vi "SR830Monitor.vi"(0 "Lock-in Reference":u16(ring) items=["Lock-in 1", "Lock-in 2", "Lock-in 3"]) -> ()   [LabVIEW 2019]
doc: "This VI is an example of storing and recovering data from the SR830 data buffers .\nDATA STORAGE RATE specifes the rate at which data is added to the data buffers .\nSCAN LENGTH specifies the approximate length of the data acquisition scan is seconds .\nPLOT GRAPH, PLOT CH 1 DATA and PLOT CH 2 DATA specify if the respective graphs will be displayed .\nAfter data storage is completed , the channel 1 and channel 2 points are downloaded from the instrument to the CH 1 POINTS and CH 2 POINTS arrays respectively . \nSince data recovered (using the SR830 receive message.vi) is in the string format , this VI requires a considerable amount of time to format the data into an array of floating point numbers . A quicker way would be to store the string in a file and use a CIN to speed up the process ."
uses:
  Utility/Monitor Communication/SR830/SR830-Cluster.ctl
  Utility/Monitor Communication/SR830/SR830-Settings-Cluster.ctl
  Global/Global Variables/Data_Display_global.vi
  Instrument_Setup.vi
  Utility/Monitor Communication/sub-vis/SR830_Open_Queue.vi
  Utility/Monitor Communication/sub-vis/SR830-2_Open_Queue.vi
  Utility/Monitor Communication/sub-vis/SR830-3_Open_Queue.vi
  Utility/Monitor Communication/sub-vis/SR830_Check_Queue.vi
panel:
  out "Sensitivity 2":i16(ring)=15 items=["2 nV", "5 nV", "10 nV", "20 nV", "50 nV", "100 nV", "200 nV", "500 nV", "1 µV", "2 µV", "5 µV", "10 µV", "20 µV", "50 µV", "100 µV", "200 µV", "500 µV", "1 mV", "2 mV", "5 mV", "10 mV", "20 mV", "50 mV", "100 mV", "200 mV", "500 mV", "1 V", ""]
  out "SR830-3 Settings":T1={"VISA"="GPIB0::17::INSTR", "Display Channel 2"={" display"=0, " ratio"=0, "output"=1}, "Display Channel 1"={" display"=0, " ratio"=0, "output"=1}, "Time constant"={"time constant\n(10 µs : 0) "=12, "slope (6 dB/oct)"=3}, "Sensitivity"={"sensitivity\n2nV/fA"=0, "dyn reserve\n(low noise:2)"=2, "ref. phase"=0.0, "automeasure"=FALSE}, "Offset - Expand."={"Expand (0: x1)"=0, "Offset/Expand Parameter (1: X)"=1, "Manual Offset (0)"=0.0}, "Reference"={"ref. source"=TRUE, "osc.harm# "=1, "osc. freq"=22.08, "osc. ampl."=5.0, "ref. trigger"=0}, "Lock In 1 sync"={"sync filter"=FALSE, "line filter\n(off:0)"=0}, "Lock In 1 input"={"input"=1, "ground"=FALSE, "couple"=TRUE}} {"Lock In 1 input"."input" items=["A", "A-B", "I (1 M gain)", "I (100 M gain)"]; "Lock In 1 sync"."line filter\n(off:0)" items=["OFF", "line", "2 x line", "both"]; "Reference"."ref. trigger" items=["sine", "pos edge", "neg edge"]; "Reference"."osc.harm#" min=1 max=19999; "Reference"."osc. ampl." format="%.3f"; "Reference"."osc. freq" format="%.3f"; "Offset - Expand."."Offset/Expand Parameter (1: X)" items=["X"=1, "Y"=2, "R"=3]; "Offset - Expand."."Expand (0: x1)" items=["x1", "x10", "x100"]; "Sensitivity"."sensitivity\n2nV/fA" items=["2 nV/fA", "5 nV/fA", "10 nV/fA", "20 nV/fA", "50 nV/fA", "100 nV/fA", "200 nV/fA", "500 nV/fA", "1 µV /pA", "2 µV/pA", "5 µV/pA", "10 µV/pA", "20 µV/pA", "50 µV/pA", "100 µV/pA", "200 µV/pA", "500 µV/pA", "1 mV/nA", "2 mV/nA", "5 mV/nA", "10 mV/nA", "20 mV/nA", "50 mV/nA", "100 mV/nA", "200 mV/nA", "500 mV/nA", "1 V/µA"]; "Sensitivity"."dyn reserve\n(low noise:2)" scale=0.0..2.0 scale format="%.2f"; "Sensitivity"."ref. phase" format="%.2f"; "Time constant"."slope (6 dB/oct)" items=["6 dB/oct", "12 dB/oct", "18 dB/oct", "24 dB/oct"]; "Time constant"."time constant\n(10 µs : 0)" items=["10 µs", "30 µs", "100 µs", "300 µs", "1 ms", "3 ms", "10 ms", "30 ms", "100 ms", "300 ms", "1 s", "3 s", "10 s", "30 s", "100 s", "300 s", "1 ks", "3 ks", "10 ks", "30 ks"]; "Display Channel 1"."output" items=["display", "X"]; "Display Channel 1"."ratio" items=["none", "aux in 1", "aux in 2"]; "Display Channel 1"."display" items=["X", "R", "X Noise", "Aux In 1", "Aux In 2"]; "Display Channel 2"."output" items=["display", "Y"]; "Display Channel 2"."ratio" items=["none", "aux in 3", "aux in 4"]; "Display Channel 2"."display" items=["Y", "@", "Y Noise", "Aux In 3", "Aux In 4"]}
  out "SR830":T2={"Lockin 1"=[], "X1-Display"=0.0, "Y1-Display"=0.0, "X1 Percent"=0.0, "X1 Overload"=FALSE, "Y1 Overload"=FALSE, "Unit X1"="nV", "Unit X2"="nV", "Unit X2a"="nV", "Unit X1a"="nV", "Sensitivity Setpoint"=26, "X1 Percent 2"=0.0, "Y1"=0.0, "X1"=0.0, "Preamp OVL"=FALSE} {"X1 Percent 2" scale=0.0..1.0; "Sensitivity Setpoint" items=["2 nV", "5 nV", "10 nV", "20 nV", "50 nV", "100 nV", "200 nV", "500 nV", "1 µV", "2 µV", "5 µV", "10 µV", "20 µV", "50 µV", "100 µV", "200 µV", "500 µV", "1 mV", "2 mV", "5 mV", "10 mV", "20 mV", "50 mV", "100 mV", "200 mV", "500 mV", "1 V", ""]; "X1 Percent" scale=0.0..1.0; "X1-Display" format="%#4_5f"}
  in  "Stopp":bool
  # "float\nground"
  # "AC\nDC"
  # "on\noff"
  # "int\next"
  # "on\noff"
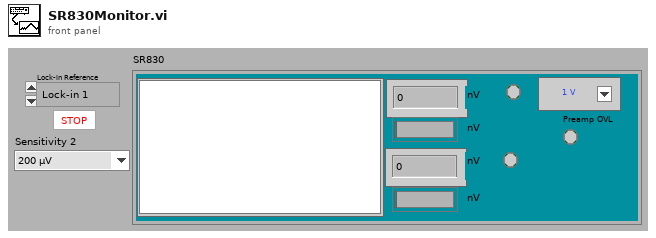
[diagram p1: front panel]
types:
  T1 = typedef "SR830-Settings-Cluster.ctl" = cluster{"VISA":refnum<visa-resource-name>, "Display Channel 2":cluster{" display":i32, " ratio":u16, "output":u16}, "Display Channel 1":cluster{" display":i32, " ratio":u16, "output":u16}, "Time constant":cluster{"time constant\n(10 µs : 0) ":i32, "slope (6 dB/oct)":i32}, "Sensitivity":cluster{"sensitivity\n2nV/fA":i32, "dyn reserve\n(low noise:2)":i16, "ref. phase":ext, "automeasure":bool}, "Offset - Expand.":cluster{"Expand (0: x1)":u16, "Offset/Expand Parameter (1: X)":u16, "Manual Offset (0)":dbl}, "Reference":cluster{"ref. source":bool, "osc.harm# ":u16, "osc. freq":ext, "osc. ampl.":ext, "ref. trigger":u16}, "Lock In 1 sync":cluster{"sync filter":bool, "line filter\n(off:0)":i32}, "Lock In 1 input":cluster{"input":u16, "ground":bool, "couple":bool}}
  T2 = typedef "SR830-Cluster.ctl" = cluster{"Lockin 1":dbl[][], "X1-Display":dbl, "Y1-Display":dbl, "X1 Percent":dbl, "X1 Overload":bool, "Y1 Overload":bool, "Unit X1":string, "Unit X2":string, "Unit X2a":string, "Unit X1a":string, "Sensitivity Setpoint":i16, "X1 Percent 2":dbl, "Y1":dbl, "X1":dbl, "Preamp OVL":bool}
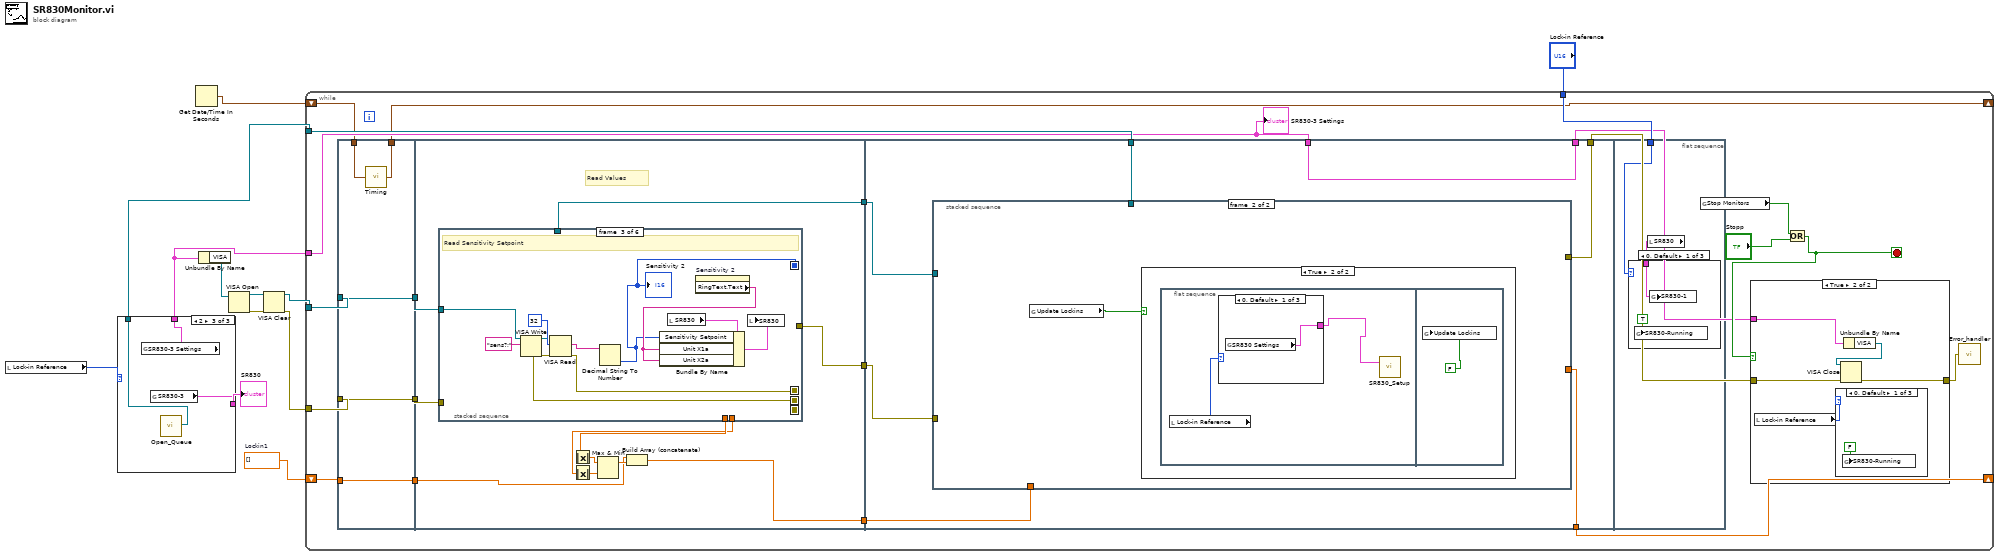
[diagram p0: block diagram]
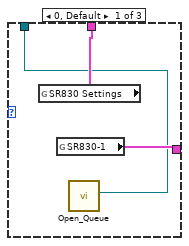
[diagram p2: hidden frame]
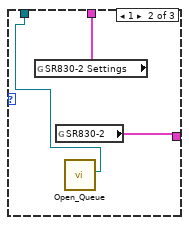
[diagram p3: hidden frame]
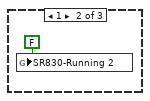
[diagram p5: hidden frame]
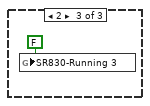
[diagram p6: hidden frame]
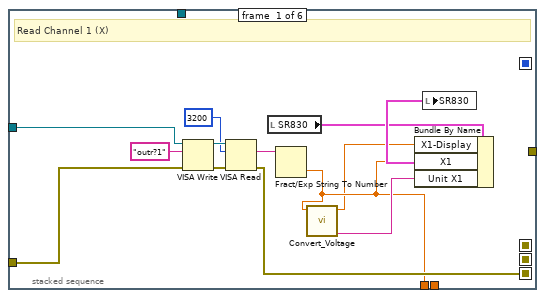
[diagram p7: hidden frame]
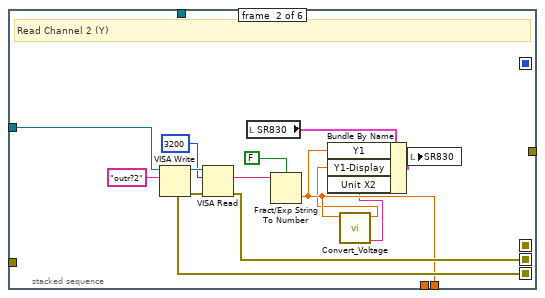
[diagram p8: hidden frame]
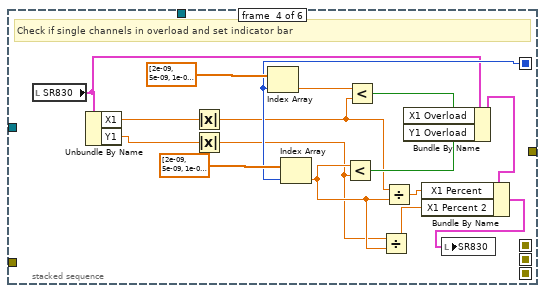
[diagram p9: hidden frame]
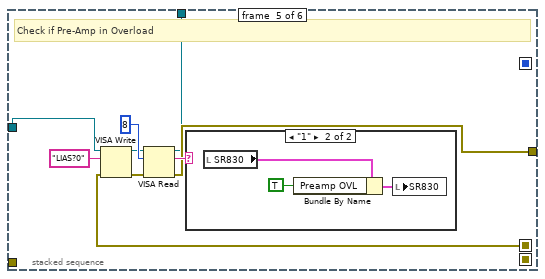
[diagram p10: hidden frame]
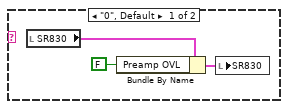
[diagram p11: hidden frame]
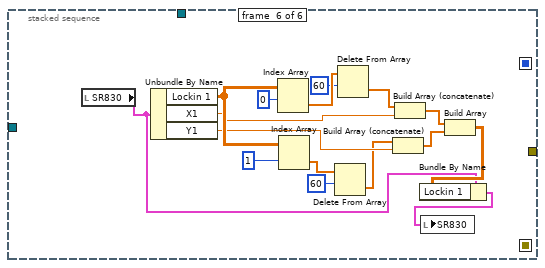
[diagram p12: hidden frame]
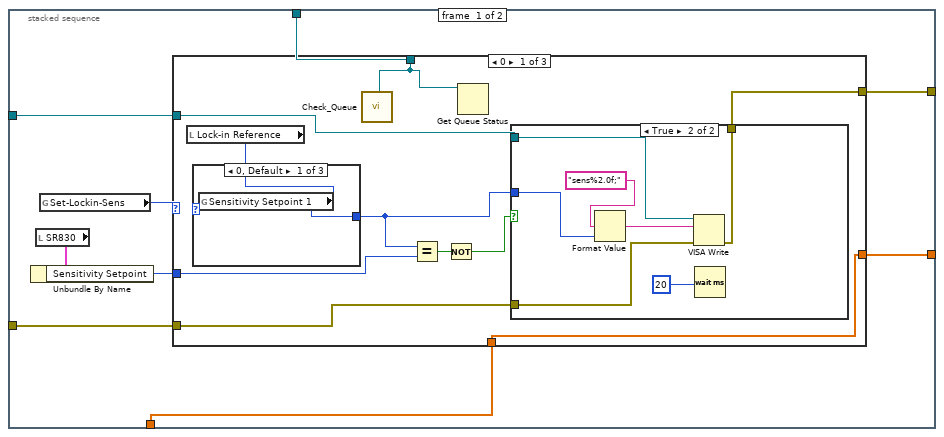
[diagram p13: hidden frame]
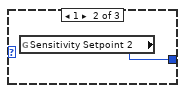
[diagram p14: hidden frame]
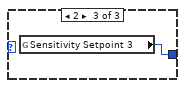
[diagram p15: hidden frame]
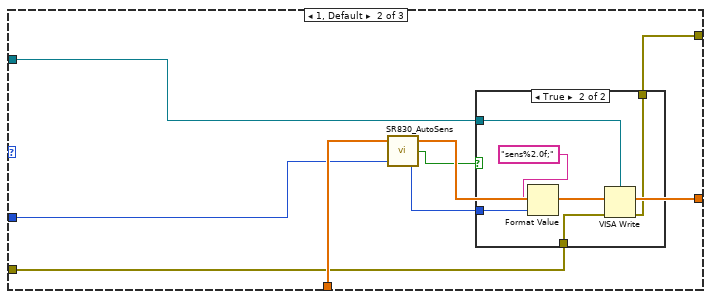
[diagram p17: hidden frame]
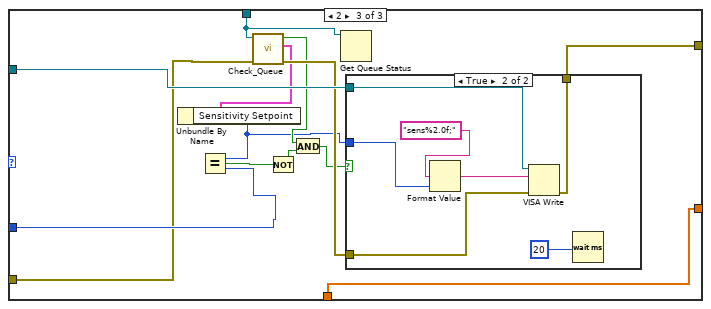
[diagram p19: hidden frame]
diagram:
  w12 = dbl[] []  # Lockin1
  n1 = local read "Lock-in Reference"() -> (w4:u16)
  n2 = case shown="2" w4 {
    tunnel: [w15 w18 w21] -> w5
    tunnel: [w14 w17 w20] -> w3
    tunnel: [w13 w16 w19] -> w2
    frame 0, Default {
      n3 = global read "Instrument_Setup.vi" "SR830 Settings"() -> (w14:T1)
      n4 = global read "Data_Display_global.vi" "SR830-1"() -> (w15:T2)
      n5 = call-poly "Open_Queue.vi"() -> ("queue out"=w13:refnum<queue>)  [unwired: 10 in, 1 out]
    }
    frame 1 {
      n6 = global read "Instrument_Setup.vi" "SR830-2 Settings"() -> (w17:T1)
      n7 = global read "Data_Display_global.vi" "SR830-2"() -> (w18:T2)
      n8 = call-poly "Open_Queue.vi"() -> ("queue out"=w16:refnum<queue>)  [unwired: 10 in, 1 out]
    }
    frame 2 {
      n9 = global read "Instrument_Setup.vi" "SR830-3 Settings"() -> (w20:T1)
      n10 = global read "Data_Display_global.vi" "SR830-3"() -> (w21:T2)
      n11 = call-poly "Open_Queue.vi"() -> ("queue out"=w19:refnum<queue>)  [unwired: 10 in, 1 out]
    }
  }
  "SR830" <- w5
  n12 = Get Date/Time In Seconds() -> (seconds since 1Jan1904=w1:timestamp)
  n13 = Unbundle By Name(w3) -> ("VISA"=w7:refnum<visa-resource-name>)
  n14 = VISA Open(VISA resource name=w7) -> (VISA resource name=w10:refnum<visa-resource-name>, error out=w11:errorcluster)  [unwired: 4 in]
  n15 = VISA Clear(VISA resource name=w10, error in (no error)=w11) -> (VISA resource name out=w9:refnum<visa-resource-name>, error out=w8:errorcluster)
  n16 = while {
    tunnel: w9 -> [w39]
    tunnel: w8 -> [w38]
    shift-right: [w34] -> _
    shift-left: w12 -> [w40]
    tunnel: w3 -> [w27]
    tunnel: w2 -> [w30]
    tunnel: "Lock-in Reference" -> [w29]
    shift-right: [w23] -> _
    shift-left: w1 -> [w22]
    stop <- w33 stop-if-true
    n17 = flat-sequence {
      tunnel: w38 -> [w54]
      tunnel: w39 -> [w55]
      tunnel: w40 -> [w56]
      tunnel: [w56] -> w26
      tunnel: [w55] -> w25
      tunnel: [w54] -> w24
      tunnel: [w53] -> w23
      tunnel: w22 -> [w52]
      tunnel: [w58] -> w37
      tunnel: [w61] -> w36
      tunnel: [w57] -> w35
      tunnel: w26 -> [w62]
      tunnel: w25 -> [w60]
      tunnel: w24 -> [w59]
      tunnel: w37 -> [w159]
      tunnel: w36 -> [w160]
      tunnel: w35 -> [w158]
      tunnel: [w157] -> w34
      tunnel: [w156] -> w32
      tunnel: w27 -> [w154]
      tunnel: w30 -> [w155]
      tunnel: [w154] -> w28
      tunnel: w29 -> [w234]
      frame #0 {
        n18 = call "Timing.vi"("start time (s)"=w52) -> ("last reading (s)"=w53:timestamp)
      }
      frame #1 {
        # "Read Values"
        n19 = stacked-sequence {
          seq-local: [w73 _ _ _ _ _] -> [_ w86 _ _ _ _]
          seq-local: [_ w85 _ _ _ _] -> [_ _ w99 _ _ _]
          seq-local: [_ _ w98 _ _ _] -> [_ _ _ _ w125 _]
          seq-local: [_ _ w96 _ _ _] -> [_ _ _ w117 _ _]
          tunnel: [w69 _ _ _ _ _] -> w65
          tunnel: [_ w83 _ _ _ _] -> w64
          tunnel: w60 -> [w72 w84 w101 _ w128 _]
          tunnel: w59 -> [w74 _ _ _ _ _]
          tunnel: [_ _ _ _ w124 _] -> w58
          tunnel: [_ _ _ _ w123 _] -> w57
          frame #0 {
            # "Read Channel 1 (X)"
            n20 = VISA Write(VISA resource name=w72, write buffer="outr?1", error in (no error)=w74) -> (VISA resource name out=w78:refnum<visa-resource-name>, error out=w79:errorcluster)  [unwired: 1 out]
            n21 = VISA Read(VISA resource name=w78, byte count=3200, error in (no error)=w79) -> (read buffer=w76:string, error out=w73:errorcluster)  [unwired: 2 out]
            n22 = local read "SR830"() -> (w71:T2)
            n23 = Fract/Exp String To Number(string=w76) -> (number=w69:dbl)  [unwired: 3 in, 1 out]
            n24 = call "Convert_Voltage.vi"("Numerisch"=w69) -> ("String"=w70:string, "Numerisch 2"=w68:dbl)  [unwired: 9 in]
            n25 = Bundle By Name(cluster=w71, "X1-Display"=w68, "X1"=w69, "Unit X1"=w70) -> (w75:T2)
            n26 = local write "SR830"(w75) -> ()
          }
          frame #1 {
            # "Read Channel 2 (Y)"
            n27 = VISA Write(VISA resource name=w84, write buffer="outr?2", error in (no error)=w86) -> (VISA resource name out=w92:refnum<visa-resource-name>, error out=w93:errorcluster)  [unwired: 1 out]
            n28 = VISA Read(VISA resource name=w92, byte count=3200, error in (no error)=w93) -> (read buffer=w87:string, error out=w85:errorcluster)  [unwired: 2 out]
            n29 = local read "SR830"() -> (w89:T2)
            n30 = Fract/Exp String To Number(use system decimal point (T)=FALSE, string=w87) -> (number=w83:dbl)  [unwired: 2 in, 1 out]
            n31 = call "Convert_Voltage.vi"("Numerisch"=w83) -> ("String"=w81:string, "Numerisch 2"=w82:dbl)  [unwired: 9 in]
            n32 = Bundle By Name(cluster=w89, "Y1"=w83, "Y1-Display"=w82, "Unit X2"=w81) -> (w90:T2)
            n33 = local write "SR830"(w90) -> ()
          }
          frame #2 {
            # "Read Sensitivity Setpoint"
            n34 = VISA Write(VISA resource name=w101, write buffer="sens?;", error in (no error)=w99) -> (VISA resource name out=w100:refnum<visa-resource-name>, error out=w105:errorcluster)  [unwired: 1 out]
            n35 = VISA Read(VISA resource name=w100, byte count=32, error in (no error)=w105) -> (read buffer=w95:string, error out=w98:errorcluster)  [unwired: 2 out]
            n36 = Decimal String To Number(string=w95) -> (number=w96:i32)  [unwired: 2 in, 1 out]
            "Sensitivity 2" <- w96
            n37 = local read "SR830"() -> (w103:T2)
            n38 = property on="Sensitivity 2" class="Ring (strict)"() -> ("RingText.Text"=w97:string)  [unwired: 2 in, 2 out]
            n39 = Bundle By Name(cluster=w103, "Sensitivity Setpoint"=w96, "Unit X1a"=w97, "Unit X2a"=w97) -> (w102:T2)
            n40 = local write "SR830"(w102) -> ()
          }
          frame #3 {
            # "Check if single channels in overload and set indicator bar"
            n41 = local read "SR830"() -> (w114:T2)
            n42 = Unbundle By Name(w114) -> ("X1"=w120:dbl, "Y1"=w118:dbl)
            n43 = Absolute Value(x=w120) -> (abs(x)=w113:dbl)
            n44 = Absolute Value(x=w118) -> (abs(x)=w111:dbl)
            n45 = Index Array(array=dbl[] [2e-09, 5e-09, 1e-08, 2e-08, 5e-08, 1e-07, 2e-07, 5e-07, 1e-06, 2e-06, 5e-06, 1e-05, 2e-05, 5e-05, 0.0001, 0.0002, 0.0005, 0.001, 0.002, 0.005, 0.01, 0.02, 0.05, 0.1, 0.2, 0.5, 1.0] ("Array"), index=w117) -> (element=w121:dbl)
            n46 = Index Array(array=dbl[] [2e-09, 5e-09, 1e-08, 2e-08, 5e-08, 1e-07, 2e-07, 5e-07, 1e-06, 2e-06, 5e-06, 1e-05, 2e-05, 5e-05, 0.0001, 0.0002, 0.0005, 0.001, 0.002, 0.005, 0.01, 0.02, 0.05, 0.1, 0.2, 0.5, 1.0] ("Array"), index=w117) -> (element=w112:dbl)
            n47 = Less?(x=w112, y=w111) -> (x < y?=w115:bool)
            n48 = Less?(x=w121, y=w113) -> (x < y?=w116:bool)
            n49 = Divide(x=w111, y=w112) -> (x/y=w108:dbl)
            n50 = Divide(x=w113, y=w112) -> (x/y=w109:dbl)
            n51 = Bundle By Name(cluster=w114, "X1 Overload"=w116, "Y1 Overload"=w115) -> (w110:T2)
            n52 = Bundle By Name(cluster=w110, "X1 Percent"=w109, "X1 Percent 2"=w108) -> (w107:T2)
            n53 = local write "SR830"(w107) -> ()
          }
          frame #4 {
            # "Check if Pre-Amp in Overload"
            n54 = VISA Write(VISA resource name=w128, write buffer="LIAS?0", error in (no error)=w125) -> (VISA resource name out=w126:refnum<visa-resource-name>, error out=w131:errorcluster)  [unwired: 1 out]
            n55 = VISA Read(VISA resource name=w126, byte count=8, error in (no error)=w131) -> (VISA resource name out=w123:refnum<visa-resource-name>, read buffer=w127:string, error out=w124:errorcluster)  [unwired: 1 out]
            n56 = case shown="\"1\"" w127 {
              frame "0", Default {
                n57 = local read "SR830"() -> (w134:T2)
                n58 = Bundle By Name(cluster=w134, "Preamp OVL"=FALSE) -> (w133:T2)
                n59 = local write "SR830"(w133) -> ()
              }
              frame "1" {
                n60 = local read "SR830"() -> (w137:T2)
                n61 = Bundle By Name(cluster=w137, "Preamp OVL"=TRUE) -> (w136:T2)
                n62 = local write "SR830"(w136) -> ()
              }
            }
          }
          frame #5 {
            n63 = local read "SR830"() -> (w139:T2)
            n64 = Unbundle By Name(w139) -> ("Lockin 1"=w153:dbl[][], "X1"=w150:dbl, "Y1"=w149:dbl)
            n65 = Index Array(array=w153, index (row)=0) -> (element=w146:dbl[])  [unwired: 1 in]
            n66 = Index Array(array=w153, index (row)=1) -> (element=w144:dbl[])  [unwired: 1 in]
            n67 = Delete From Array(array=w144, length=60) -> (deleted portion=w143:dbl[])  [unwired: 1 in, 1 out]
            n68 = Delete From Array(array=w146, length=60) -> (deleted portion=w145:dbl[])  [unwired: 1 in, 1 out]
            n69 = Build Array (concatenate)(w143, w149) -> (w148:dbl[])
            n70 = Build Array (concatenate)(w145, w150) -> (w147:dbl[])
            n71 = Build Array(w147, w148) -> (w140:dbl[][])
            n72 = Bundle By Name(cluster=w139, "Lockin 1"=w140) -> (w138:T2)
            n73 = local write "SR830"(w138) -> ()
          }
        }
        n74 = Absolute Value(x=w65) -> (abs(x)=w67:dbl)
        n75 = Absolute Value(x=w64) -> (abs(x)=w66:dbl)
        n76 = Max & Min(x=w67, y=w66) -> (max(x,y)=w63:dbl)  [unwired: 1 out]
        n77 = Build Array (concatenate)(w62, w63) -> (w61:dbl[])
      }
      frame #2 {
        n78 = stacked-sequence {
          tunnel: [w164 _] -> w157
          tunnel: w160 -> [w165 _]
          tunnel: w159 -> [w168 _]
          tunnel: w158 -> [w167 _]
          tunnel: [w166 _] -> w156
          tunnel: w155 -> [w161 _]
          frame #0 {
            n79 = local read "SR830"() -> (w163:T2)
            n80 = Unbundle By Name(w163) -> ("Sensitivity Setpoint"=w162:i16)
            n81 = global read "Instrument_Setup.vi" "Set-Lockin-Sens"() -> (w169:u16)
            n82 = case shown="0" w169 {
              tunnel: w168 -> [w179 w192 w207]
              tunnel: w167 -> [w177 w194 w218]
              tunnel: [w178 w191 w211] -> w166
              tunnel: w165 -> [w176 w198 w210]
              tunnel: [w176 w197 w210] -> w164
              tunnel: w162 -> [w173 w196 w209]
              tunnel: w161 -> [w175 _ w206]
              frame 0 {
                n83 = local read "Lock-in Reference"() -> (w174:u16)
                n84 = case shown="0, Default" w174 {
                  tunnel: [w180 w181 w182] -> w172
                  frame 0, Default {
                    n85 = global read "Data_Display_global.vi" "Sensitivity Setpoint 1"() -> (w180:i32)
                  }
                  frame 1 {
                    n86 = global read "Data_Display_global.vi" "Sensitivity Setpoint 2"() -> (w181:i32)
                  }
                  frame 2 {
                    n87 = global read "Data_Display_global.vi" "Sensitivity Setpoint 3"() -> (w182:i32)
                  }
                }
                n88 = call-poly "Check_Queue.vi"("queue"=w175) -> ()  [unwired: 7 in, 3 out]
                n89 = Equal?(x=w172, y=w173) -> (x = y?=w171:bool)
                n90 = Not(x=w171) -> (.not. x?=w170:bool)
                n91 = Get Queue Status(queue=w175) -> ()  [unwired: 2 in, 8 out]
                n92 = case shown="True" w170 {
                  tunnel: w172 -> [_ w190]
                  tunnel: [w183 w189] -> w178
                  tunnel: w179 -> [w183 w186]
                  tunnel: w177 -> [_ w185]
                  frame False {
                  }
                  frame True {
                    n93 = Format Value(format string="sens%2.0f;", value (0)=w190) -> (output string=w188:string)  [unwired: 1 in]
                    n94 = VISA Write(VISA resource name=w185, write buffer=w188, error in (no error)=w186) -> (error out=w189:errorcluster)  [unwired: 2 out]
                    n95 = Wait (ms)(milliseconds to wait=20) -> ()  [unwired: 1 out]
                  }
                }
              }
              frame 1, Default {
                n96 = call "SR830_AutoSens.vi"("Sensitivity"=w196, "Data in"=w198) -> ("Sensitivity Out"=w193:i32, "Set Sensitivity"=w195:bool, "Data out"=w197:dbl[])  [unwired: 1 in]
                n97 = case shown="True" w195 {
                  tunnel: w194 -> [_ w203]
                  tunnel: w193 -> [_ w202]
                  tunnel: w192 -> [w199 w201]
                  tunnel: [w199 w200] -> w191
                  frame False {
                  }
                  frame True {
                    n98 = Format Value(format string="sens%2.0f;", value (0)=w202) -> (output string=w205:string)  [unwired: 1 in]
                    n99 = VISA Write(VISA resource name=w203, write buffer=w205, error in (no error)=w201) -> (error out=w200:errorcluster)  [unwired: 2 out]
                  }
                }
              }
              frame 2 {
                n100 = call-poly "Check_Queue.vi"("error in (no error)"=w207, "queue"=w206) -> ("error out"=w217:errorcluster, "SR830"=w216:T2, "New Entries?"=w213:bool)  [unwired: 6 in]
                n101 = Unbundle By Name(w216) -> ("Sensitivity Setpoint"=w208:i16)
                n102 = Equal?(x=w208, y=w209) -> (x = y?=w215:bool)
                n103 = Not(x=w215) -> (.not. x?=w214:bool)
                n104 = And(x=w213, y=w214) -> (x .and. y?=w212:bool)
                n105 = Get Queue Status(queue=w206) -> ()  [unwired: 2 in, 8 out]
                n106 = case shown="True" w212 {
                  tunnel: w208 -> [_ w226]
                  tunnel: [w219 w225] -> w211
                  tunnel: w217 -> [w219 w222]
                  tunnel: w218 -> [_ w221]
                  frame False {
                  }
                  frame True {
                    n107 = Format Value(format string="sens%2.0f;", value (0)=w226) -> (output string=w224:string)  [unwired: 1 in]
                    n108 = VISA Write(VISA resource name=w221, write buffer=w224, error in (no error)=w222) -> (error out=w225:errorcluster)  [unwired: 2 out]
                    n109 = Wait (ms)(milliseconds to wait=20) -> ()  [unwired: 1 out]
                  }
                }
              }
            }
          }
          frame #1 {
            n110 = global read "Instrument_Setup.vi" "Update Lockins"() -> (w227:bool)
            n111 = case shown="True" w227 {
              frame False {
              }
              frame True {
                n112 = flat-sequence {
                  frame #0 {
                    n113 = local read "Lock-in Reference"() -> (w228:u16)
                    n114 = case shown="0, Default" w228 {
                      tunnel: [w230 w231 w232] -> w229
                      frame 0, Default {
                        n115 = global read "Instrument_Setup.vi" "SR830 Settings"() -> (w230:T1)
                      }
                      frame 1 {
                        n116 = global read "Instrument_Setup.vi" "SR830-2 Settings"() -> (w231:T1)
                      }
                      frame 2 {
                        n117 = global read "Instrument_Setup.vi" "SR830-3 Settings"() -> (w232:T1)
                      }
                    }
                    n118 = call "SR830_Setup.vi"("SR830 Settings Cluster"=w229) -> ()  [unwired: 2 in]
                  }
                  frame #1 {
                    n119 = global write "Instrument_Setup.vi" "Update Lockins"(FALSE) -> ()
                  }
                }
              }
            }
          }
        }
      }
      frame #3 {
        n120 = local read "SR830"() -> (w235:T2)
        n121 = case shown="0, Default" w234 {
          tunnel: w235 -> [w237 w239 w241]
          frame 0, Default {
            n122 = global write "Data_Display_global.vi" "SR830-Running"(TRUE) -> ()
            n123 = global write "Data_Display_global.vi" "SR830-1"(w237) -> ()
          }
          frame 1 {
            n124 = global write "Data_Display_global.vi" "SR830-Running 2"(TRUE) -> ()
            n125 = global write "Data_Display_global.vi" "SR830-2"(w239) -> ()
          }
          frame 2 {
            n126 = global write "Data_Display_global.vi" "SR830-Running 3"(TRUE) -> ()
            n127 = global write "Data_Display_global.vi" "SR830-3"(w241) -> ()
          }
        }
      }
    }
    n128 = global read "Data_Display_global.vi" "Stop Monitors"() -> (w42:bool)
    n129 = Or(x=w42, y="Stopp") -> (x .or. y?=w33:bool)
    n130 = case shown="True" w33 {
      tunnel: w32 -> [w43 w47]
      tunnel: [w43 w46] -> w31
      tunnel: w28 -> [_ w45]
      frame False {
      }
      frame True {
        n131 = local read "Lock-in Reference"() -> (w44:u16)
        n132 = case shown="0, Default" w44 {
          frame 0, Default {
            n133 = global write "Data_Display_global.vi" "SR830-Running"(FALSE) -> ()
          }
          frame 1 {
            n134 = global write "Data_Display_global.vi" "SR830-Running 2"(FALSE) -> ()
          }
          frame 2 {
            n135 = global write "Data_Display_global.vi" "SR830-Running 3"(FALSE) -> ()
          }
        }
        n136 = Unbundle By Name(w45) -> ("VISA"=w48:refnum<visa-resource-name>)
        n137 = VISA Close(VISA resource name=w48, error in (no error)=w47) -> (error out=w46:errorcluster)
      }
    }
    n138 = call "Error_handler.vi"("error constant"=w31) -> ()
    "SR830-3 Settings" <- w27
  }
